vi "Text Array to String.vi"(10 "List Data":i32[](array[ring]) items=["CURR", "VOLT"]) -> (2 "Result String":string)   [LabVIEW 2023, in "Agilent B2900 Series.lvlib"]
doc: "Parse a text array into a comma separated string which can be recognized by SCPI commands"
uses:
  Agilent B2900 Series.lvlib
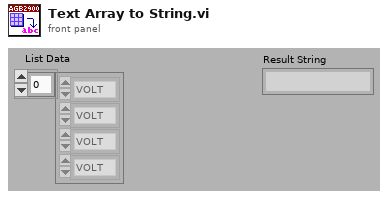
[diagram p1: front panel]
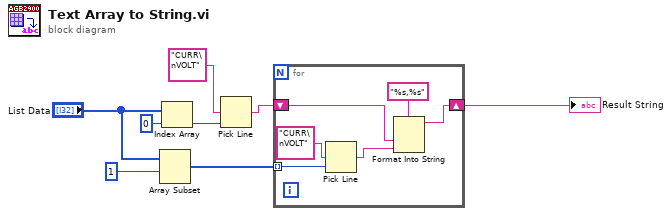
[diagram p0: block diagram]
diagram:
  n1 = Array Subset(array="List Data", index=1) -> (w7:i32[])  [unwired: 1 in]
  n2 = Index Array(array="List Data", index=0) -> (element=w3:i32)
  n3 = Pick Line(multi-line string="CURR\nVOLT" ("format string"), line index=w3) -> (output string=w2:string)  [unwired: 1 in]
  n4 = for {
    tunnel: w7 -> [w11] mode=indexing
    shift-right: [w14] -> w8
    shift-left: w2 -> [w13]
    n5 = Pick Line(multi-line string="CURR\nVOLT" ("format string"), line index=w11) -> (output string=w9:string)  [unwired: 1 in]
    n6 = Format Into String(format string="%s,%s", w13, w9) -> (resulting string=w14:string)  [unwired: 2 in, 1 out]
  }
  "Result String" <- w8
